vi "Read Spectra from Data Object.vi"(8 "error in (no error)":errorcluster, 10 "component":T7=32 items=["Magnitude^2"=37, "Magnitude"=32, "Phase"=33, "Real"=34, "Imaginary"=35, "Coherence"=36, "Unknown"=99], 11 "Y (Complex) (N Ch) in":refnum<class "Y (Complex) (N Ch).lvclass">) -> (0 "error out":errorcluster, 1 "spectra info":T1[](array[typedef]) {"x-axis units" items=["Time (s)"=0, "Frequency-CB (Hz)"=1, "Frequency-CPB (Hz)"=1248, "Frequency-Arbitrary (Hz)"=2357, "Quefrency (s)"=2, "Revolutions (rev)"=3, "Order"=4, "Speed (RPM)"=11, "Speed (rad/s)"=21, "Index"=65535]; "weighting filter" items=["Linear", "A-weighting", "B-weighting", "C-weighting", "ITU-R 468-4", "Dolby", "CCITT", "C-message", "Wb", "Wc", "Wd", "We", "Wf", "Wh", "Wj", "Wk", "Wm", "AES17 20 kHz lowpass", "AES17 40 kHz lowpass", "AES17 20 kHz highpass", "AES17 40 kHz highpass"]; "dB reference [EU]" format="%.2f"; "engineering units" items=["custom..."=0, "V"=1, "A"=21, "C"=30, "pC"=31, "s"=32, "-"=29, "Pa"=2, "N"=20, "g"=3, "m/s^2"=4, "m/s"=5, "m"=6, "mm/s"=12, "mm"=13, "micron/s"=14, "micron"=15, "in/s^2"=7, "in/s"=8, "in"=9, "mil/s"=10, "mil"=11, "rad/s^2"=16, "rad/s"=17, "rad"=18, "deg/s^2"=26, "deg/s"=27, "deg"=28, "RPM"=22, "cycle/s^2"=23, "Hz"=24, "cycle"=25, "strain"=19]; "spectral info"."window" items=["None "=0, "Hanning"=1, "Hamming"=2, "Blackman-Harris"=3, "Exact Blackman"=4, "Blackman"=5, "Flat Top"=6, "4 Term B-Harris "=7, "7 Term B-Harris"=8, "Low Sidelobe"=9, "Force - Exponential"=10, "Gaussian"=62]}, 2 "spectra":cluster{"x0":dbl, "dx":dbl, "Y":dbl[]}[](array[cluster]), 3 "Y (Complex) (N Ch) out":refnum<class "Y (Complex) (N Ch).lvclass">, 4 "global attributes":variant)   [LabVIEW 2017, in "Y (Complex) (N Ch).lvclass"]
uses:
  <vilib>/addons/_NISVFA/_Shared subVIs/Data Objects/Y (Complex) (DBL)/Y (Complex) (N Ch).lvclass
  C:/Program Files (x86)/National Instruments/LabVIEW 2017/vi.lib/addons/_NISVFA/_Shared subVIs/Data Objects/Data/Data.lvclass
  <vilib>/addons/_NISVFA/_Shared subVIs/Controls/NI Spectrum Component.ctl
  <vilib>/addons/_NISVFA/_Shared subVIs/Controls/svc_Spectrum Info.ctl
  <vilib>/addons/_NISVFA/_Shared subVIs/Controls/svc_X-Axis Units.ctl
  <vilib>/addons/_NISVFA/_Shared subVIs/Controls/svc_Spectrum Type.ctl
  <vilib>/addons/_NISVFA/_Shared subVIs/Controls/svc_Engineering Units Text Ring.ctl
  <vilib>/addons/_NISVFA/_Shared subVIs/Controls/svc_Weighting Filter Text Ring.ctl
  <vilib>/addons/_NISVFA/_Shared subVIs/Controls/svc_Complimentary Spectrum Units.ctl
  <vilib>/addons/_NISVFA/_Shared subVIs/Data Objects/Data/Data.lvclass/Data.ctl
  <vilib>/addons/_NISVFA/_Shared subVIs/Data Objects/Y (Complex) (DBL)/Y (Complex) (N Ch).lvclass/Y (Complex) (N Ch).ctl
  <vilib>/addons/_NISVFA/_Shared subVIs/Common/sv_Get NI Property Name String.vi
  <vilib>/addons/_NISVFA/_Shared subVIs/Common/sv_Get SV Property Name String.vi
  <vilib>/addons/_NISVFA/_Shared subVIs/Common/svc_Spectrum Units.vi
  <vilib>/addons/_NISVFA/_Shared subVIs/Spectrum Info/sfva_Set SV Info in Spectrum Info Description.vi
  <vilib>/addons/_NISVFA/_Shared subVIs/Common/svc_Get Weighting Enum and Labels.vi
  <vilib>/addons/_NISVFA/_Shared subVIs/Common/svc_Unit Label Lexical Class.vi
  <vilib>/addons/_NISVFA/_Shared subVIs/Common/svc_Engineering Units to Unit Label.vi
  <vilib>/addons/_NISVFA/_Shared subVIs/Common/svc_Format Value (DBL).vi
  <vilib>/addons/_NISVFA/_Shared subVIs/Data Objects/Data/Data.lvclass
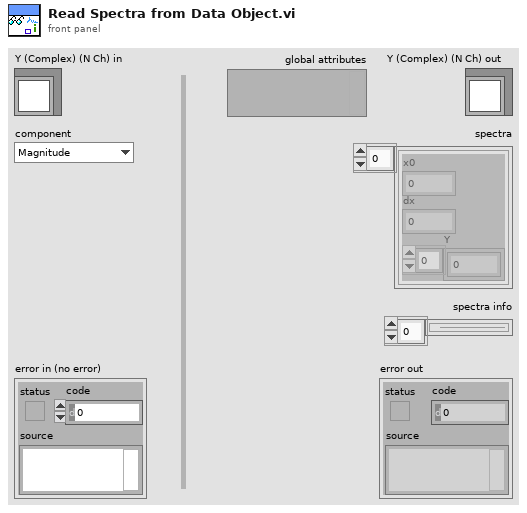
[diagram p1: front panel]
types:
  T1 = typedef "svc_Spectrum Info.ctl" = cluster{"channel name":string, "description":string, "x-axis units":T2, "spectral info":cluster{"spectrum type":T3, "linear/dB":enum16{"linear", "dB"}, "window":u16, "window size":i32, "FFT size":i32}, "engineering units":T4, "custom label":string, "dB reference [EU]":dbl, "peak units":enum16{"rms", "peak", "peak-peak"}, "weighting filter":T5, "spectral density?":bool, "unit label":string, "spectrum skewed?":bool, "complimentary spectrum units":T6}
  T2 = typedef "svc_X-Axis Units.ctl" = u16
  T3 = typedef "svc_Spectrum Type.ctl" = enum16{"FFT Spectrum [complex]", "Amplitude [Magnitude]", "Power [Magnitude^2]", "Cross Spectrum [complex]", "Frequency Response [Complex]"}
  T4 = typedef "svc_Engineering Units Text Ring.ctl" = u16
  T5 = typedef "svc_Weighting Filter Text Ring.ctl" = u16
  T6 = typedef "svc_Complimentary Spectrum Units.ctl" = enum16{"none", "radians", "degrees", "cycles", "imaginary"}
  T7 = typedef "NI Spectrum Component.ctl" = u16
  T8 = cluster{"Y":cdb[], "channel attributes":variant}[]
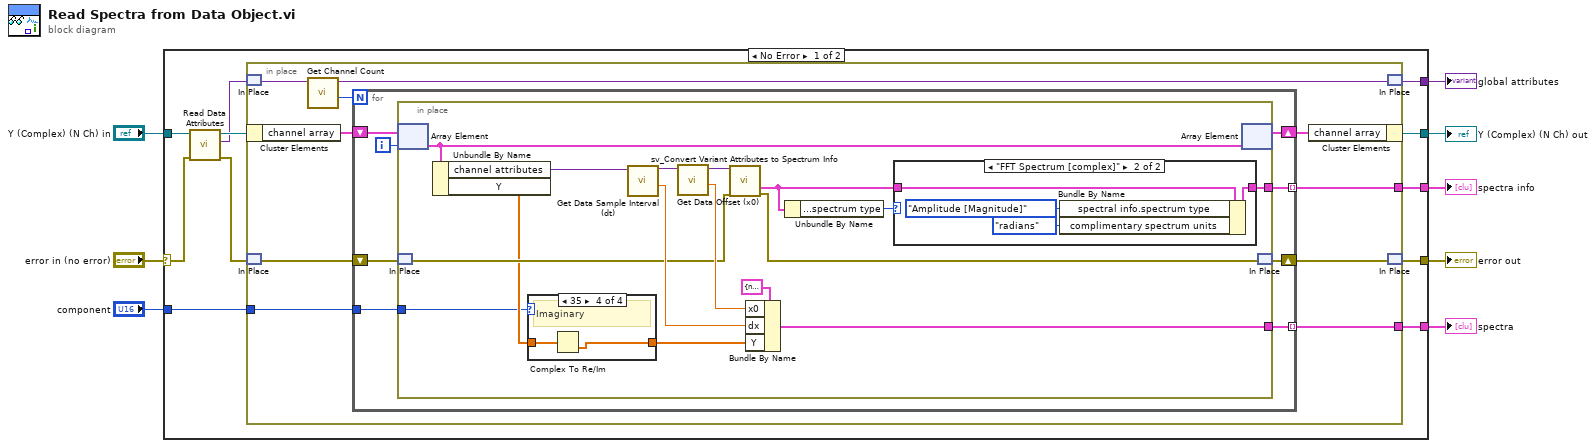
[diagram p0: block diagram]
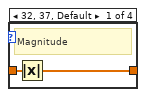
[diagram p2: hidden frame]
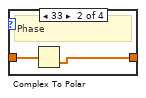
[diagram p3: hidden frame]
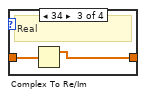
[diagram p4: hidden frame]
diagram:
  n1 = case shown="No Error" "error in (no error)" {
    selector: "error in (no error)" -> [w16 w68]
    tunnel: [w14 w68] -> w1
    tunnel: [w19 w67] -> w7
    tunnel: "Y (Complex) (N Ch) in" -> [w18 w67]
    tunnel: [w10 _] -> w3
    tunnel: [w13 _] -> w5
    tunnel: [w12 _] -> w4
    tunnel: "component" -> [w9 _]
    frame No Error {
      n2 = call <vilib>:"Read Data Attributes.vi"("error in (no error)"=w16, "Data in"=w18) -> ("error out"=w15:errorcluster, "data attributes"=w11:variant, "Data out"=w17:refnum<class "Y (Complex) (N Ch).lvclass">)  [unwired: 7 in]
      n3 = in-place {
        in-place-border: [w25] -> w13
        in-place-border: [w24] -> w12
        in-place-border: w9 -> [w20]
        n4 = in-place-match #1(w11) -> (w23:variant)
        n5 = in-place-cluster #2(w17) -> ("channel array"=w29:T8)
        n6 = in-place-match #3(w15) -> (w27:errorcluster)
        n7 = call <vilib>:"Get Channel Count.vi"("variant in"=w23) -> ("number of channels"=w21:i32, "variant out"=w22:variant)  [unwired: 9 in]
        n8 = for {
          N: w21 -> [_]
          shift-right: [w36] -> w28
          shift-left: w29 -> [w37]
          shift-right: [w33] -> w26
          shift-left: w27 -> [w34]
          tunnel: [w32] -> w25 mode=indexing
          tunnel: [w31] -> w24 mode=indexing
          tunnel: w20 -> [w30]
          i -> [w35]
          n9 = in-place {
            in-place-border: [w41] -> w32
            in-place-border: [w44] -> w31
            in-place-border: w30 -> [w38]
            n10 = in-place-array #4(w37, w35) -> (w53:cluster{"Y":cdb[], "channel attributes":variant})
            n11 = in-place-match #5(w34) -> (w46:errorcluster)
            n12 = Unbundle By Name(w53) -> ("channel attributes"=w51:variant, "Y"=w40:cdb[])
            n13 = case shown="35" w38 {
              tunnel: w40 -> [w55 w57 w59 w61]
              tunnel: [w54 w56 w58 w60] -> w39
              frame 32, 37, Default {
                # "Magnitude"
                n14 = Absolute Value(x=w55) -> (abs(x)=w54:dbl[])
              }
              frame 33 {
                # "Phase"
                n15 = Complex To Polar(r * e^(i*theta)=w57) -> (theta=w56:dbl[])  [unwired: 1 out]
              }
              frame 34 {
                # "Real"
                n16 = Complex To Re/Im(x + iy=w59) -> (x=w58:dbl[])  [unwired: 1 out]
              }
              frame 35 {
                # "Imaginary"
                n17 = Complex To Re/Im(x + iy=w61) -> (y=w60:dbl[])  [unwired: 1 out]
              }
            }
            n18 = call <vilib>:"Get Data Sample Interval (dt).vi"("variant in"=w51) -> ("dt [s]"=w50:dbl, "variant out"=w52:variant)  [unwired: 9 in]
            n19 = call <vilib>:"Get Data Offset (x0).vi"("data attributes"=w52) -> ("x0"=w49:dbl, "data attributes"=w48:variant)  [unwired: 9 in]
            n20 = call <vilib>:"sv_Convert Variant Attributes to Spectrum Info.vi"("variant attributes"=w48, "error in"=w46) -> ("spectrum info"=w42:T1, "error out"=w45:errorcluster)  [unwired: 11 in, 1 out]
            n21 = Bundle By Name(cluster=cluster{"x0":dbl, "dx":dbl, "Y":dbl[]} {"x0"=nan, "dx"=nan, "Y"=[nan]} ("power spectrum [dB EU]"), "x0"=w49, "dx"=w50, "Y"=w39) -> (w44:cluster{"x0":dbl, "dx":dbl, "Y":dbl[]})
            n22 = Unbundle By Name(w42) -> ("spectral info.spectrum type"=w43:T3)
            n23 = case shown="\"FFT Spectrum [complex]\"" w43 {
              tunnel: [w62 w63] -> w41
              tunnel: w42 -> [w62 w64]
              frame Default {
              }
              frame "FFT Spectrum [complex]" {
                n24 = Bundle By Name(cluster=w64, "spectral info.spectrum type"=svc_Spectrum_Type."Amplitude [Magnitude]", "complimentary spectrum units"=svc_Complimentary_Spectrum_Units."radians") -> (w63:T1)
              }
            }
            n25 = in-place-array #4(w53) -> (w36:T8)  [unwired: 1 out]
            n26 = in-place-match #5(w45) -> (w33:errorcluster)
          }
        }
        n27 = in-place-cluster #2("channel array"=w28) -> (w19:refnum<class "Y (Complex) (N Ch).lvclass">)
        n28 = in-place-match #1(w22) -> (w10:variant)
        n29 = in-place-match #3(w26) -> (w14:errorcluster)
      }
    }
    frame Error {
    }
  }
  "error out" <- w1
  "Y (Complex) (N Ch) out" <- w7
  "global attributes" <- w3
  "spectra" <- w4
  "spectra info" <- w5
